vi "Select HDF5 Dialog.vi"   [LabVIEW 2017]
doc: "Displays a dialog prompting the user to select a dataset, datatype,\n or group from an HDF5 file."
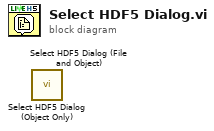
[diagram p0: block diagram]
diagram:
  n1 = call <vilib>:"Select HDF5 Dialog (Object Only).vi"() -> ()  [unwired: 11 in, 5 out]
  n2 = call <vilib>:"Select HDF5 Dialog (File and Object).vi"() -> ()  [unwired: 10 in, 6 out]
